vi "Timing_Main_Pulse_Delay.vi"(8 "Source of Ticks":tag="/Dev1/100kHzTimebase" caption="20MHz-Clock", 9 "Trigger Source":tag="/Dev1/PFI9" caption="Signal in", 10 "Counter(s)":tag="Dev1/ctr0" caption="Delay Out", 11 "Delay / [us]":i32) -> (0 "error out":errorcluster, 3 "task out":refnum<k21>)   [LabVIEW 2009]
uses:
  <vilib>/DAQmx/configure/trigger.llb/DAQmx Start Trigger (Digital Edge).vi
  <vilib>/DAQmx/create/channels.llb/DAQmx Create Channel (CO-Pulse Generation-Ticks).vi
  Program Files/National Instruments/LabVIEW 2009/resource/objmgr/daqmx.rc
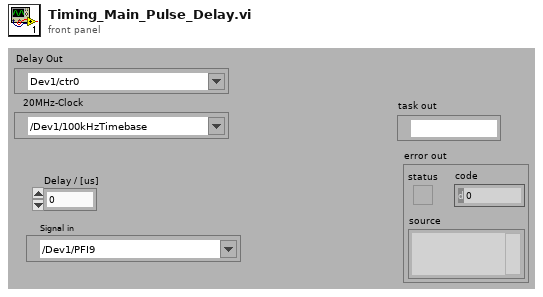
[diagram p1: front panel]
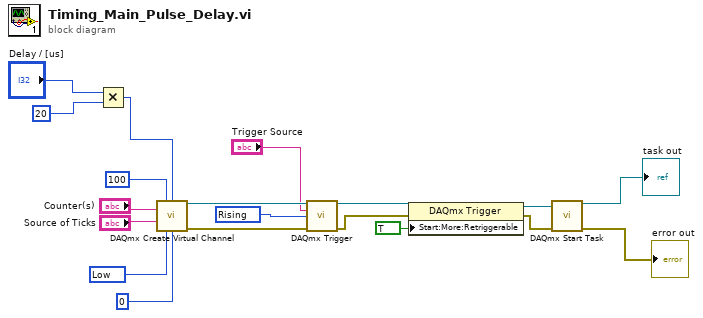
[diagram p0: block diagram]
diagram:
  w13 = 10280 items=["Rising"=10280, "Falling"=10171] ("Trigger Edge")
  w12 = 10214 items=["High"=10192, "Low"=10214] ("Idle State")
  n1 = Multiply(x="Delay / [us]", y=20) -> (x*y=w3:i32)
  n2 = call-poly <vilib>:"DAQmx Create Virtual Channel.vi"("high ticks"=u32 100 ("High Ticks"), "low ticks"=w3, "counter"="Counter(s)", "source of ticks"="Source of Ticks", "idle state"=w12, "initial delay"=u32 0 ("Initial Delay")) -> ("task out"=w16:refnum<k21>, "error out"=w15:errorcluster)  [unwired: 3 in, 5 out]
  n3 = call-poly <vilib>:"DAQmx Trigger.vi"("task/channels in"=w16, "source"="Trigger Source", "edge"=w13, "error in"=w15) -> ("task out"=w9:refnum<k21>, "error out"=w8:errorcluster)  [unwired: 10 out]
  n4 = property class="DAQmx Trigger"(reference=w9, error in=w8, "Start:More:Retriggerable"=TRUE) -> (reference out=w7:refnum<k21>, error out=w6:errorcluster)
  n5 = call <vilib>:"DAQmx Start Task.vi"("task/channels in"=w7, "error in"=w6) -> ("task out"=→"task out":refnum<k21>, "error out"=→"error out":errorcluster)  [unwired: 12 out]
